vi "Task Config.vi"(8 "error in":errorcluster) -> (0 "error out":errorcluster, 3 "task out":refnum<k21>)   [LabVIEW 2009]
uses:
  <vilib>/DAQmx/create/channels.llb/DAQmx Create Channel (AI-Current-Basic).vi
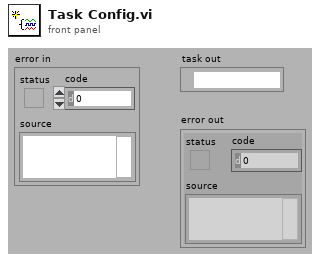
[diagram p1: front panel]
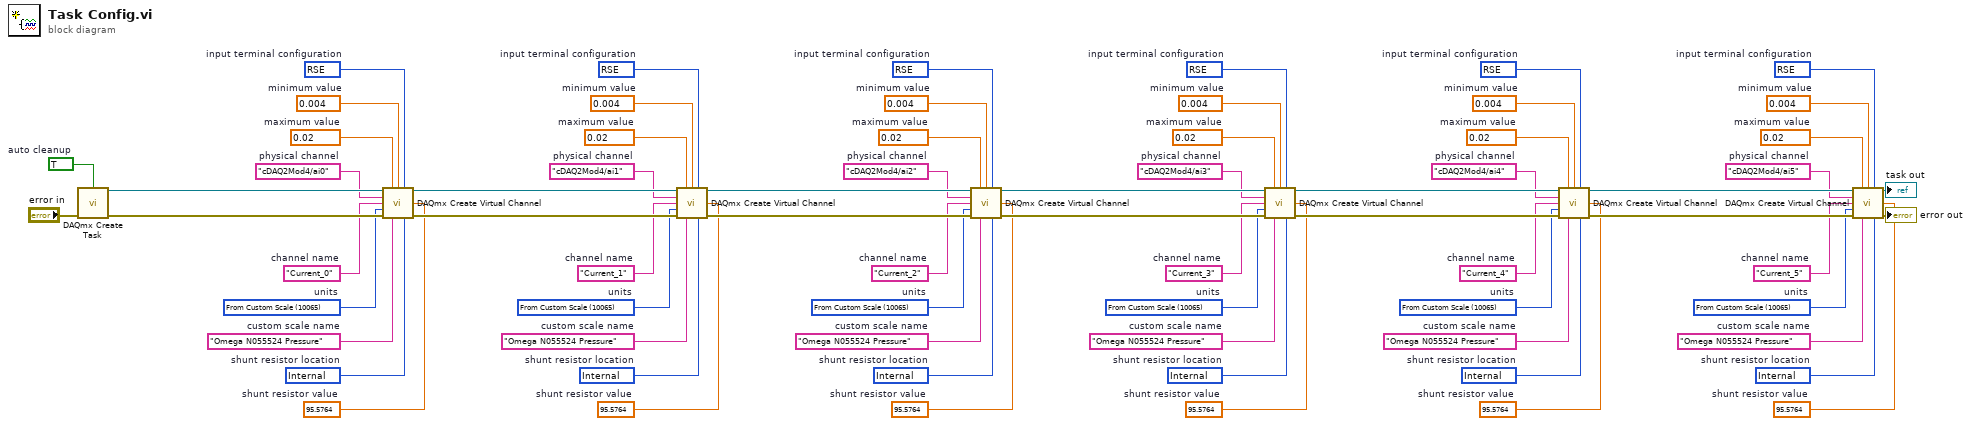
[diagram p0: block diagram]
diagram:
  w1 = 10083 items=["default"=-1, "RSE"=10083, "NRSE"=10078, "Differential"=10106, "Pseudodifferential"=12529]  # input terminal configuration
  w2 = 10065 items=["Amps"=10342, "From Custom Scale"=10065]  # units
  w3 = 95.5764  # shunt resistor value
  w4 = 10200 items=["Internal"=10200, "External"=10167]  # shunt resistor location
  w5 = "Current_5"  # channel name
  w8 = "Omega N055524 Pressure"  # custom scale name
  w9 = 0.004  # minimum value
  w10 = 0.02  # maximum value
  w11 = "cDAQ2Mod4/ai5"  # physical channel
  w13 = 10083 items=["default"=-1, "RSE"=10083, "NRSE"=10078, "Differential"=10106, "Pseudodifferential"=12529]  # input terminal configuration
  w14 = 10065 items=["Amps"=10342, "From Custom Scale"=10065]  # units
  w15 = 95.5764  # shunt resistor value
  w16 = 10200 items=["Internal"=10200, "External"=10167]  # shunt resistor location
  w17 = "Current_4"  # channel name
  w19 = "Omega N055524 Pressure"  # custom scale name
  w20 = 0.004  # minimum value
  w21 = 0.02  # maximum value
  w22 = "cDAQ2Mod4/ai4"  # physical channel
  w24 = 10083 items=["default"=-1, "RSE"=10083, "NRSE"=10078, "Differential"=10106, "Pseudodifferential"=12529]  # input terminal configuration
  w25 = 10065 items=["Amps"=10342, "From Custom Scale"=10065]  # units
  w26 = 95.5764  # shunt resistor value
  w27 = 10200 items=["Internal"=10200, "External"=10167]  # shunt resistor location
  w28 = "Current_3"  # channel name
  w30 = "Omega N055524 Pressure"  # custom scale name
  w31 = 0.004  # minimum value
  w32 = 0.02  # maximum value
  w33 = "cDAQ2Mod4/ai3"  # physical channel
  w35 = 10083 items=["default"=-1, "RSE"=10083, "NRSE"=10078, "Differential"=10106, "Pseudodifferential"=12529]  # input terminal configuration
  w36 = 10065 items=["Amps"=10342, "From Custom Scale"=10065]  # units
  w37 = 95.5764  # shunt resistor value
  w38 = 10200 items=["Internal"=10200, "External"=10167]  # shunt resistor location
  w39 = "Current_2"  # channel name
  w41 = "Omega N055524 Pressure"  # custom scale name
  w42 = 0.004  # minimum value
  w43 = 0.02  # maximum value
  w44 = "cDAQ2Mod4/ai2"  # physical channel
  w46 = 10083 items=["default"=-1, "RSE"=10083, "NRSE"=10078, "Differential"=10106, "Pseudodifferential"=12529]  # input terminal configuration
  w47 = 10065 items=["Amps"=10342, "From Custom Scale"=10065]  # units
  w48 = 95.5764  # shunt resistor value
  w49 = 10200 items=["Internal"=10200, "External"=10167]  # shunt resistor location
  w50 = "Current_1"  # channel name
  w52 = "Omega N055524 Pressure"  # custom scale name
  w53 = 0.004  # minimum value
  w54 = 0.02  # maximum value
  w55 = "cDAQ2Mod4/ai1"  # physical channel
  w57 = 10083 items=["default"=-1, "RSE"=10083, "NRSE"=10078, "Differential"=10106, "Pseudodifferential"=12529]  # input terminal configuration
  w58 = 10065 items=["Amps"=10342, "From Custom Scale"=10065]  # units
  w59 = 95.5764  # shunt resistor value
  w60 = 10200 items=["Internal"=10200, "External"=10167]  # shunt resistor location
  w61 = "Current_0"  # channel name
  w63 = "Omega N055524 Pressure"  # custom scale name
  w64 = 0.004  # minimum value
  w65 = 0.02  # maximum value
  w66 = "cDAQ2Mod4/ai0"  # physical channel
  w68 = TRUE  # auto cleanup
  n1 = call <vilib>:"DAQmx Create Task.vi"("auto cleanup"=w68, "error in"="error in") -> ("task out"=w67:refnum<k21>, "error out"=w69:errorcluster)  [unwired: 12 in]
  n2 = call-poly <vilib>:"DAQmx Create Virtual Channel.vi"("task in"=w67, "maximum value"=w65, "minimum value"=w64, "input terminal configuration"=w57, "physical channels"=w66, "name to assign"=w61, "external shunt resistor value"=w59, "units"=w58, "error in"=w69, "custom scale name"=w63, "shunt resistor location"=w60) -> ("task out"=w56:refnum<k21>, "error out"=w62:errorcluster)  [unwired: 3 in]
  n3 = call-poly <vilib>:"DAQmx Create Virtual Channel.vi"("task in"=w56, "maximum value"=w54, "minimum value"=w53, "input terminal configuration"=w46, "physical channels"=w55, "name to assign"=w50, "external shunt resistor value"=w48, "units"=w47, "error in"=w62, "custom scale name"=w52, "shunt resistor location"=w49) -> ("task out"=w45:refnum<k21>, "error out"=w51:errorcluster)  [unwired: 3 in]
  n4 = call-poly <vilib>:"DAQmx Create Virtual Channel.vi"("task in"=w45, "maximum value"=w43, "minimum value"=w42, "input terminal configuration"=w35, "physical channels"=w44, "name to assign"=w39, "external shunt resistor value"=w37, "units"=w36, "error in"=w51, "custom scale name"=w41, "shunt resistor location"=w38) -> ("task out"=w34:refnum<k21>, "error out"=w40:errorcluster)  [unwired: 3 in]
  n5 = call-poly <vilib>:"DAQmx Create Virtual Channel.vi"("task in"=w34, "maximum value"=w32, "minimum value"=w31, "input terminal configuration"=w24, "physical channels"=w33, "name to assign"=w28, "external shunt resistor value"=w26, "units"=w25, "error in"=w40, "custom scale name"=w30, "shunt resistor location"=w27) -> ("task out"=w23:refnum<k21>, "error out"=w29:errorcluster)  [unwired: 3 in]
  n6 = call-poly <vilib>:"DAQmx Create Virtual Channel.vi"("task in"=w23, "maximum value"=w21, "minimum value"=w20, "input terminal configuration"=w13, "physical channels"=w22, "name to assign"=w17, "external shunt resistor value"=w15, "units"=w14, "error in"=w29, "custom scale name"=w19, "shunt resistor location"=w16) -> ("task out"=w12:refnum<k21>, "error out"=w18:errorcluster)  [unwired: 3 in]
  n7 = call-poly <vilib>:"DAQmx Create Virtual Channel.vi"("task in"=w12, "maximum value"=w10, "minimum value"=w9, "input terminal configuration"=w1, "physical channels"=w11, "name to assign"=w5, "external shunt resistor value"=w3, "units"=w2, "error in"=w18, "custom scale name"=w8, "shunt resistor location"=w4) -> ("task out"=→"task out":refnum<k21>, "error out"=→"error out":errorcluster)  [unwired: 3 in]
